vi "filterWheel.vi"() -> ()   [LabVIEW 2017]
panel:
  out "number":i32
  out "read buffer":string
  in  "filter index":u8(ring)=1 items=["ch_BFP"=1, "ch_Cerulean"=2, "ch_GFP"=3, "ch_mOrange"=4, "ch_mCherry"=5, "ch_Ceruleanfor505nm"=7, "ch_mNeptune"=6, "ch_mNeptune2"=8, "empty (CAREFUL)"=9]
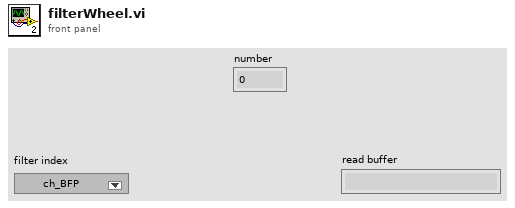
[diagram p1: front panel]
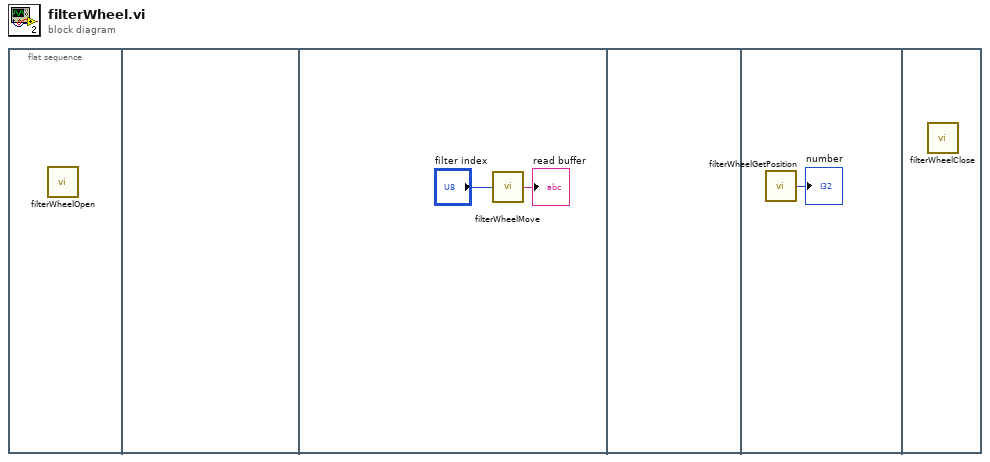
[diagram p0: block diagram]
diagram:
  n1 = flat-sequence {
    frame #0 {
      n2 = call "filterWheelOpen.vi"() -> ()  [unwired: 12 in]
    }
    frame #1 {
    }
    frame #2 {
      n3 = call "filterWheelMove.vi"("filter index"="filter index") -> ("read buffer"=→"read buffer":string)
    }
    frame #3 {
    }
    frame #4 {
      n4 = call "filterWheelGetPosition.vi"() -> ("number"=→"number":i32)  [unwired: 1 in]
    }
    frame #5 {
      n5 = call "filterWheelClose.vi"() -> ()  [unwired: 12 in]
    }
  }
